vi "Configure AUX Output.vi"(8 "Error In (no error)":errorcluster, 9 "Voltage (0.0)":dbl format="%.2f", 10 "Output (0: AUX 1)":u16(ring) items=["AUX 1", "AUX 2"], 11 "VISA Resource Name":refnum<visa-resource-name>) -> (0 "Error Out":errorcluster, 3 "VISA Resource Name Out":refnum<visa-resource-name>)   [LabVIEW 2010, in "Stanford Research 844.lvlib"]
doc: "This VI configures AUX output."
uses:
  <instrlib>/Stanford Research 844/Stanford Research 844.lvlib
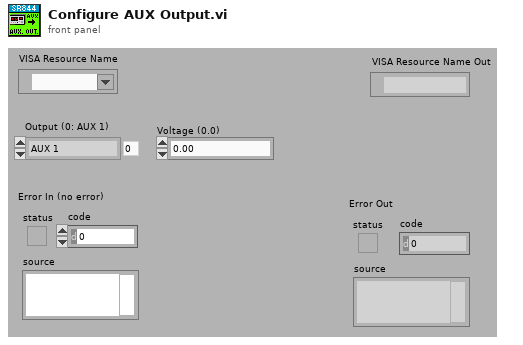
[diagram p1: front panel]
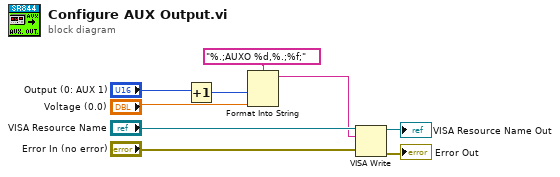
[diagram p0: block diagram]
diagram:
  n1 = Increment(x="Output (0: AUX 1)") -> (x+1=w2:u16)
  n2 = Format Into String(format string="%.;AUXO %d,%.;%f;", w2, "Voltage (0.0)") -> (resulting string=w1:string)  [unwired: 2 in, 1 out]
  n3 = VISA Write(VISA resource name="VISA Resource Name", write buffer=w1, error in (no error)="Error In (no error)") -> (VISA resource name out=→"VISA Resource Name Out":refnum<visa-resource-name>, error out=→"Error Out":errorcluster)  [unwired: 1 out]
